vi "Waveplatecontrol_stepscan2.vi"() -> ()   [LabVIEW 2015]
uses:
  <vilib>/DAQmx/write.llb/DAQmx Write (Analog DBL 1Chan 1Samp).vi
  <vilib>/DAQmx/miscellaneous.llb/DAQmx Fill In Error Info.vi
  <vilib>/DAQmx/create/channels.llb/DAQmx Create Channel (AO-Voltage-Basic).vi
  <vilib>/Analysis/1siggen.llb/Ramp Pattern by Delta.vi
  subvi/Newport ESP301/Newport ESP301.lvlib
  <vilib>/Analysis/NI_AALBase.lvlib
panel:
  in  "StepSize":i32=128
  in  "ms2wait":u32
  in  "Boolean":bool
  out "a":waveform(dbl)(graph)={"t0"=timestamp(3620209335.8073797 s since 1904-01-01), "dt"=1.0, "Y"=[nan]}
  out "Waveform Chart":dbl(graph)=5.25341140860948
  out "x*y":dbl=nan
  in  "physical channels":tag="Dev3/ao1"
  out "DAC error":errorcluster
  out "ESP error":errorcluster={"status"=TRUE, "code"=-1073807343, "source"="VISA Open in Newport ESP301.lvlib:Initialize.vi->main002.vi"}
  out "run?":bool
  in  "set_vel":bool
  in  "velocity [fs/s]":dbl=667.128190396304
  in  "vel_mm":dbl caption="velocity [deg/s]"
  out "meas. velocity":dbl=nan
  in  "stop":bool
  out "output voltage":dbl=nan
  in  "start":bool
  in  "go2p1":bool
  out "position [mm]":dbl=nan
  in  "p2 [mm]":dbl=2.0
  in  "p1 [mm]":dbl
  in  "interpolate output":bool
  in  "Delta2 [fs]":dbl=6671.281903963041
  in  "Delta1 [fs]":dbl=-6671.281903963041
  in  "Reference [mm]":dbl=1.0
  in  "Axis (1)":i32=2 min=1 max=3
  in  "Serial Link (RS232)":enum16{"RS232", "USB"}(ring)
  in  "VISA resource name":refnum<visa-resource-name>="COM9"
  in  "main_close":bool
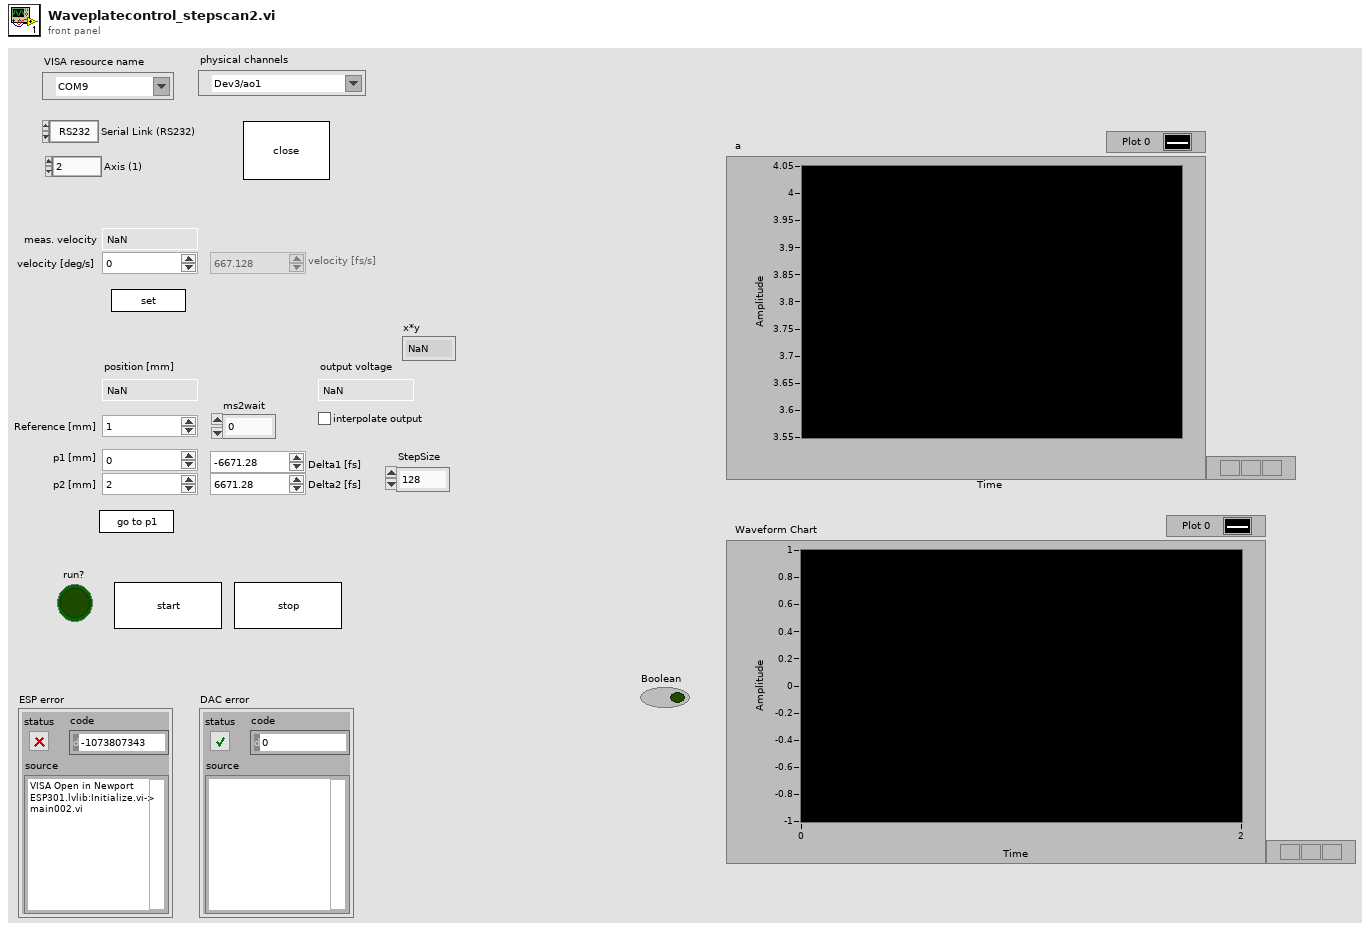
[diagram p1: front panel]
types:
  T1 = cluster{"dev1_data":refnum<queue>, "dev2_data":refnum<queue>}
  T2 = cluster{"dev1_cmd":refnum<queue>, "dev2_cmd":refnum<queue>}
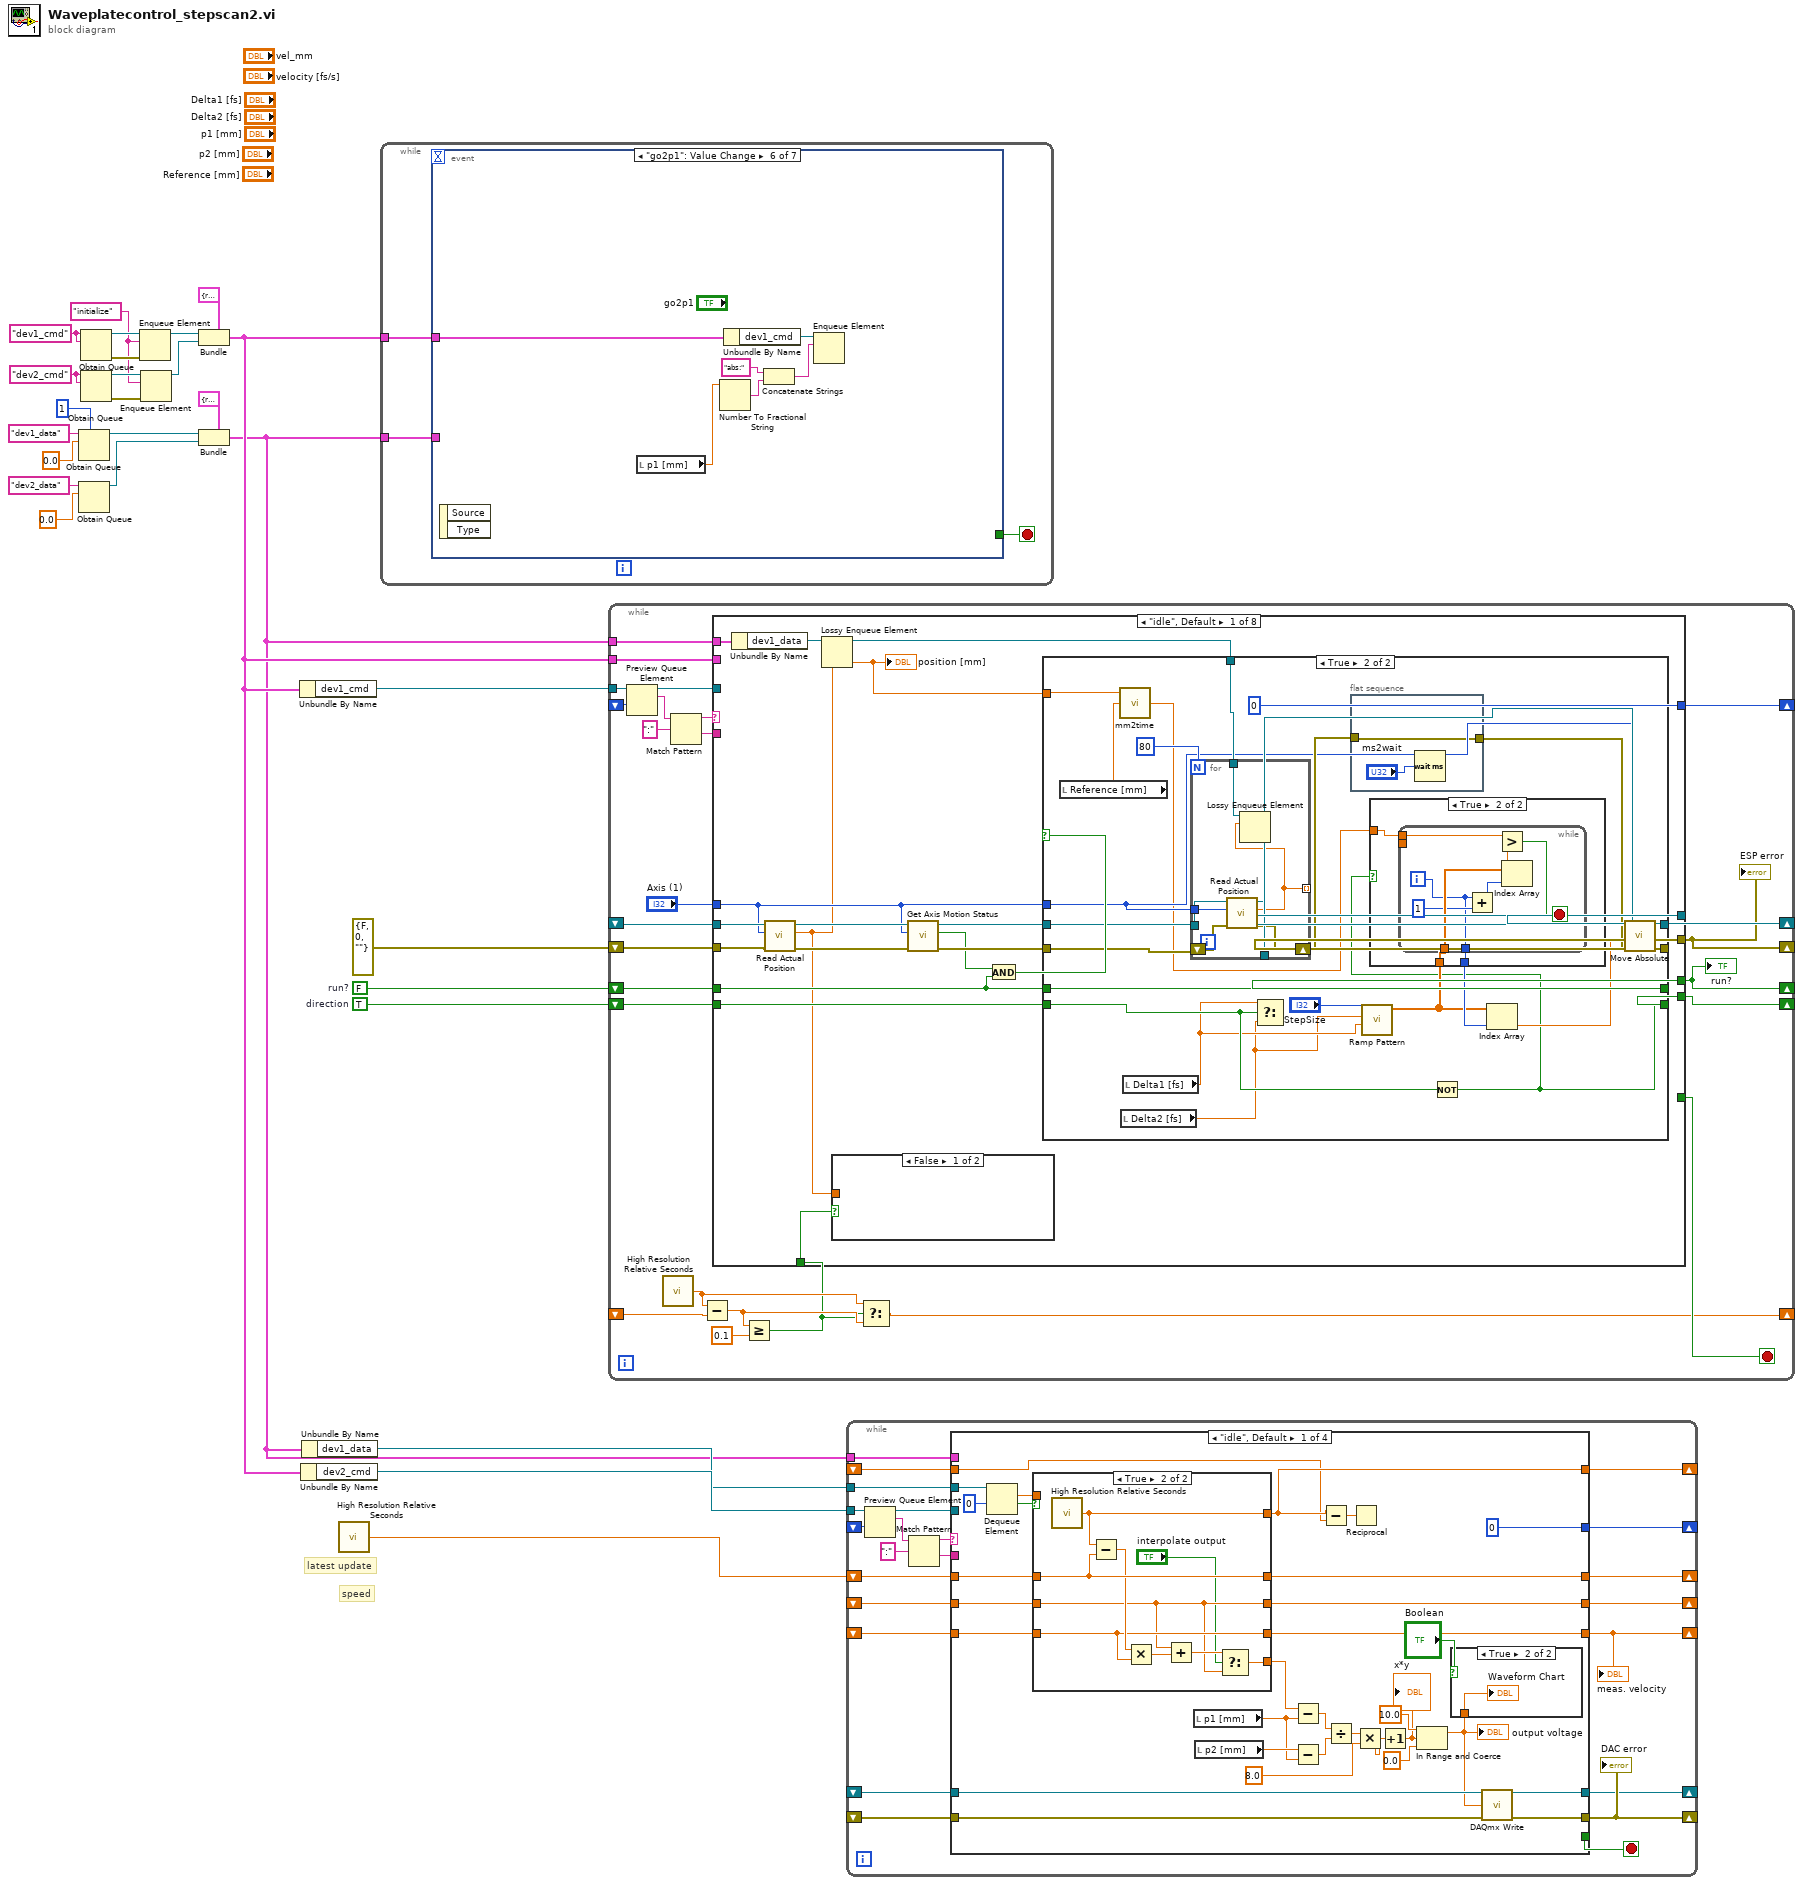
[diagram p0: block diagram]
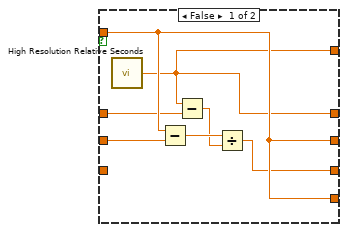
[diagram p3: hidden frame]
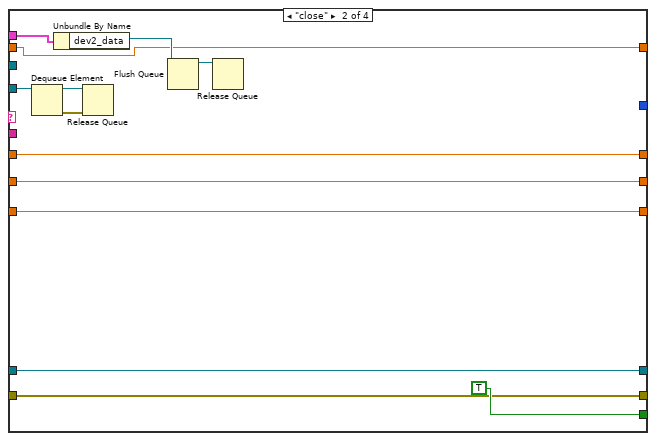
[diagram p4: hidden frame]
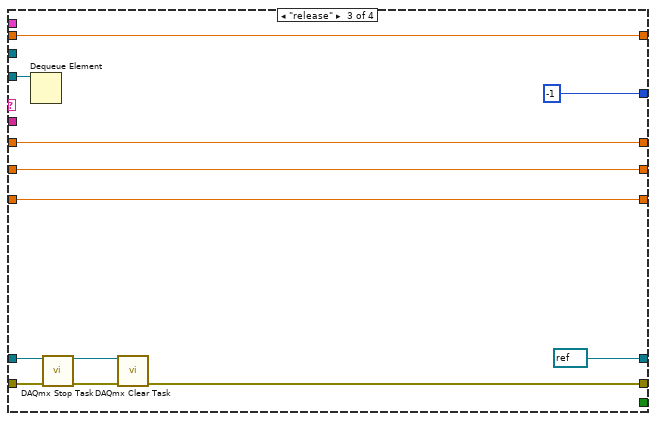
[diagram p5: hidden frame]
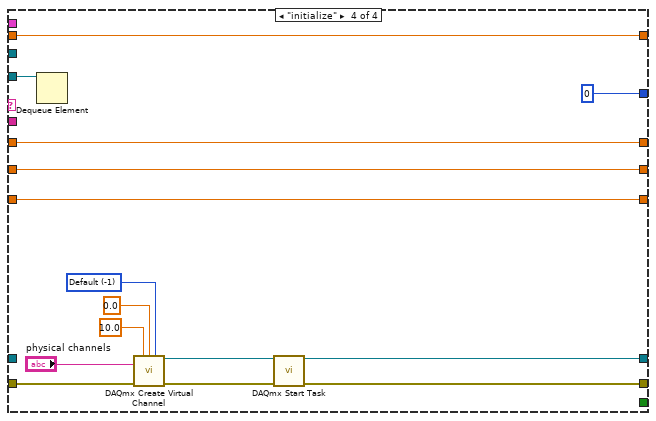
[diagram p6: hidden frame]
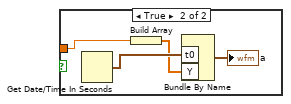
[diagram p7: hidden frame]
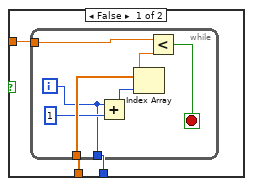
[diagram p9: hidden frame]
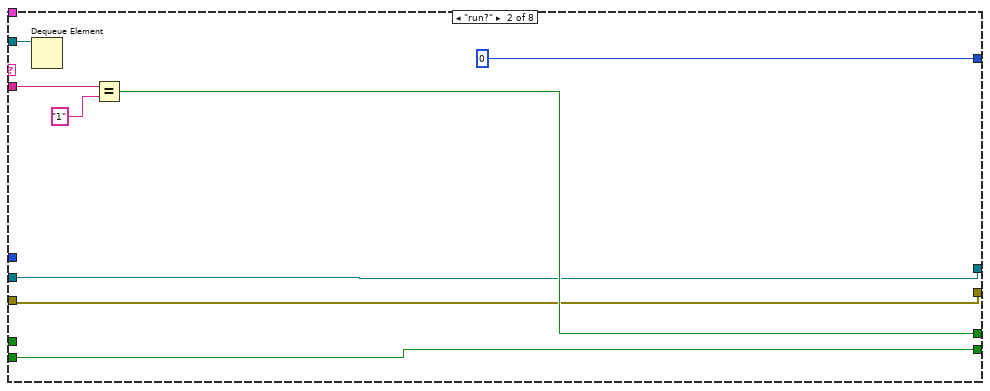
[diagram p10: hidden frame]
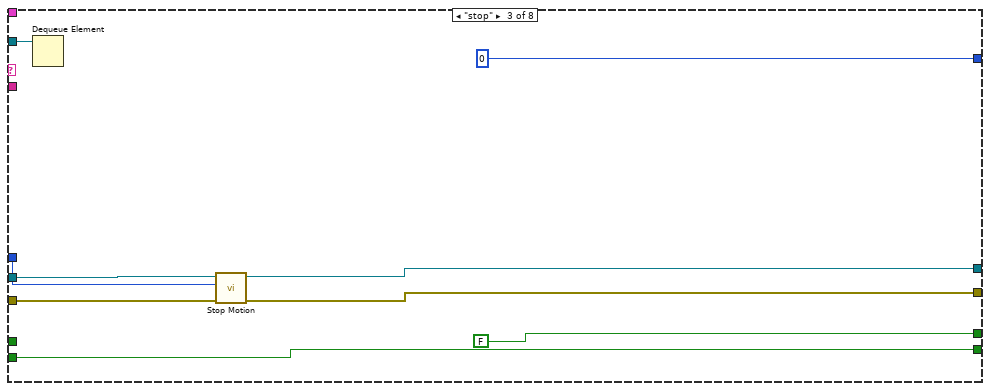
[diagram p11: hidden frame]
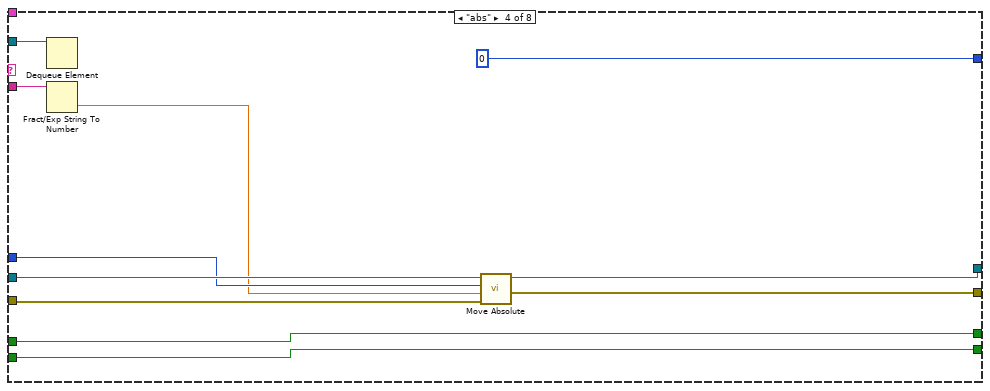
[diagram p12: hidden frame]
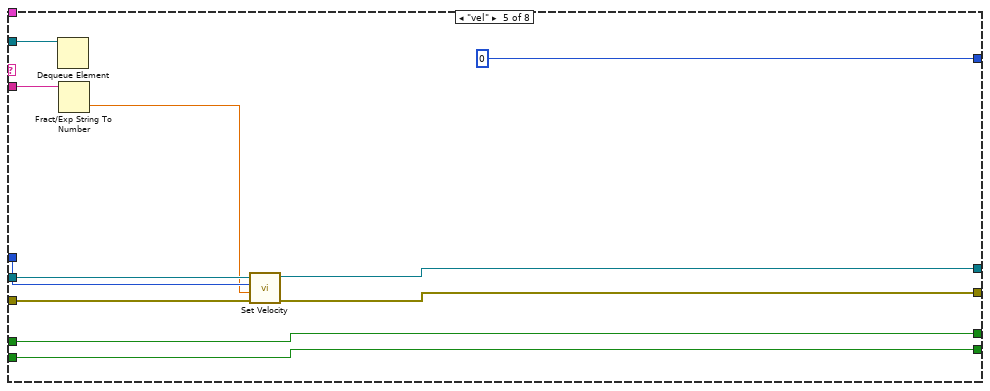
[diagram p13: hidden frame]
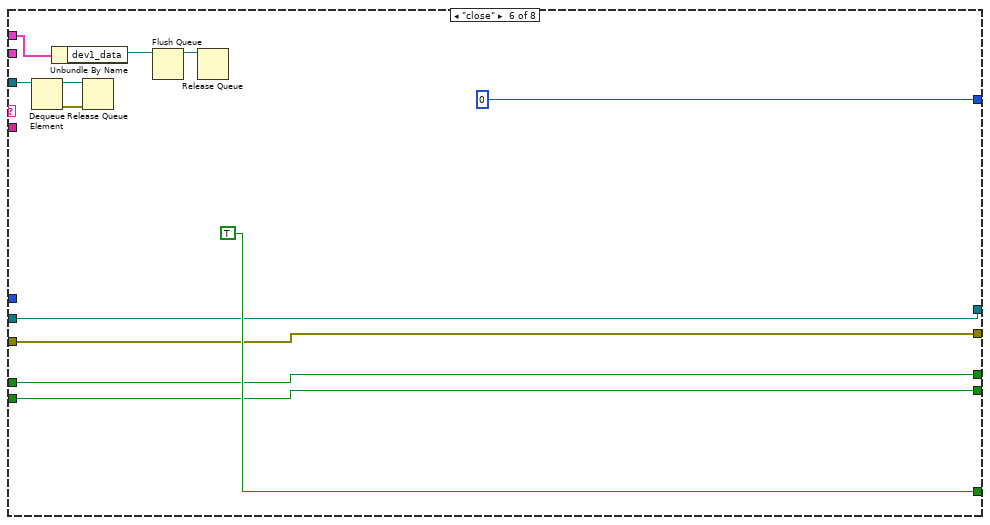
[diagram p14: hidden frame]
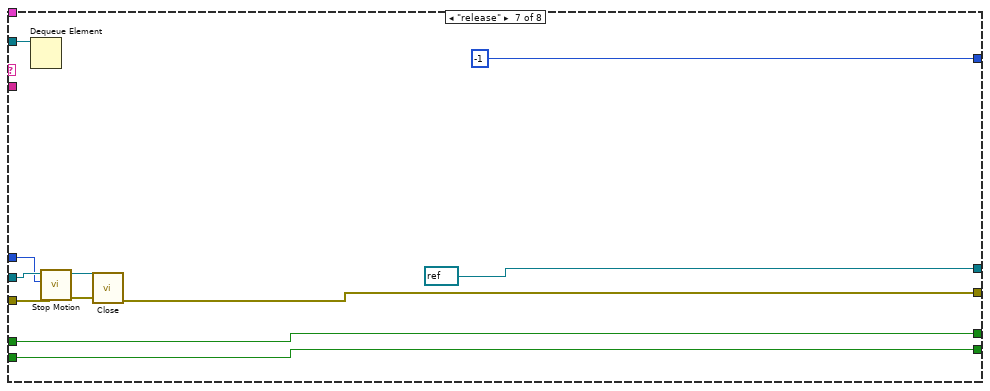
[diagram p15: hidden frame]
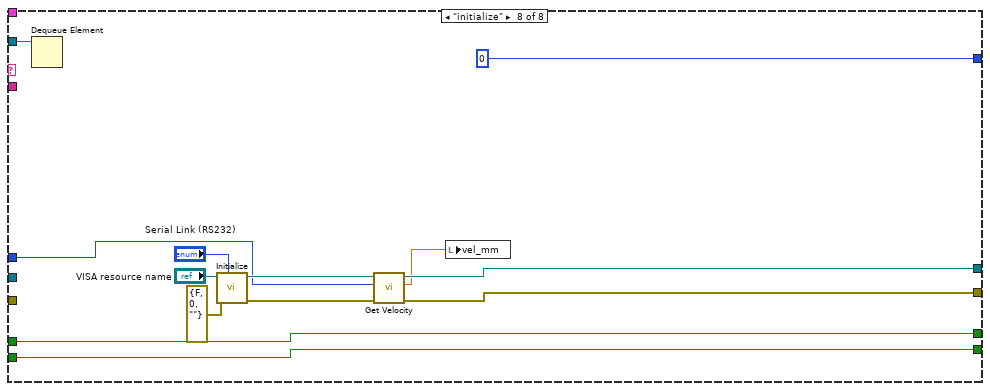
[diagram p16: hidden frame]
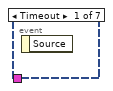
[diagram p17: hidden frame]
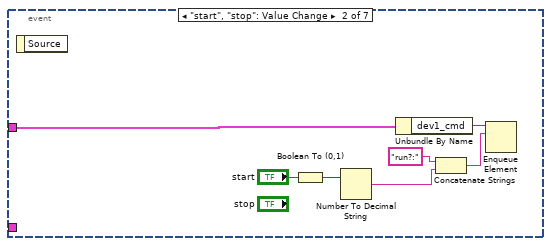
[diagram p18: hidden frame]
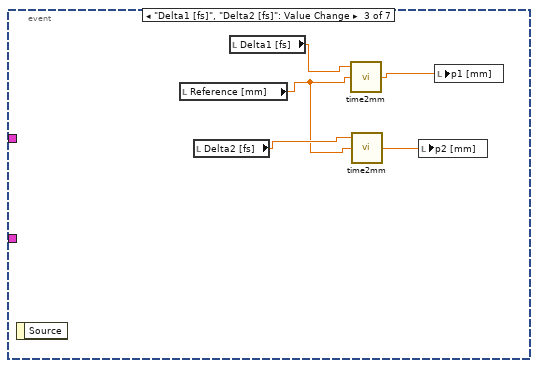
[diagram p19: hidden frame]
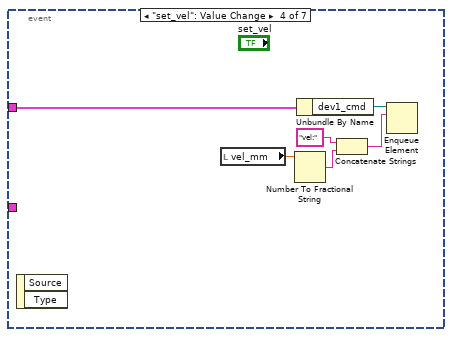
[diagram p20: hidden frame]
diagram:
  w1 = TRUE  # direction
  w4 = FALSE  # run?
  w15 = "dev2_cmd" ("name (unnamed)")
  w21 = "initialize" ("element")
  w16 = "dev1_cmd" ("name (unnamed)")
  # "speed"
  # "latest update"
  n1 = Obtain Queue(max queue size (-1, unlimited)=1, name (unnamed)="dev1_data", element data type=0.0) -> (queue out=w12:refnum<queue>)  [unwired: 2 in, 2 out]
  n2 = Obtain Queue(name (unnamed)="dev2_data", element data type=0.0) -> (queue out=w11:refnum<queue>)  [unwired: 3 in, 2 out]
  n3 = Obtain Queue(name (unnamed)=w16, element data type=w16) -> (queue out=w27:refnum<queue>, error out=w26:errorcluster)  [unwired: 3 in, 1 out]
  n4 = Obtain Queue(name (unnamed)=w15, element data type=w15) -> (queue out=w22:refnum<queue>, error out=w23:errorcluster)  [unwired: 3 in, 1 out]
  n5 = Enqueue Element(queue=w27, element=w21, error in (no error)=w26) -> (queue out=w24:refnum<queue>)  [unwired: 1 in, 2 out]
  n6 = Enqueue Element(queue=w22, element=w21, error in (no error)=w23) -> (queue out=w20:refnum<queue>)  [unwired: 1 in, 2 out]
  n7 = Bundle(cluster=T2 {"dev1_cmd"=refnum, "dev2_cmd"=refnum}, "dev1_cmd"=w24, "dev2_cmd"=w20) -> (w8:T2)
  n8 = Bundle(cluster=T1 {"dev1_data"=refnum, "dev2_data"=refnum}, "dev1_data"=w12, "dev2_data"=w11) -> (w2:T1)
  n9 = Unbundle By Name(w8) -> ("dev1_cmd"=w17:refnum<queue>)
  n10 = Unbundle By Name(w8) -> ("dev2_cmd"=w7:refnum<queue>)
  n11 = Unbundle By Name(w2) -> ("dev1_data"=w6:refnum<queue>)
  n12 = call <vilib>:"High Resolution Relative Seconds.vi"() -> ("relative seconds"=w5:dbl)
  n13 = while {
    tunnel: w8 -> [w30]
    tunnel: w2 -> [w29]
    stop <- w28 stop-if-true
    n14 = event shown="[5] \"go2p1\": Value Change" {
      selector: _ -> [_ _ _ _ _ _ _]
      dyn-events: _ -> [_ _ _ _ _ _ _]
      timeout: _ -> [_ _ _ _ _ _ _]
      tunnel: w30 -> [_ w34 _ w44 _ w62 w65]
      tunnel: w29 -> [_ _ _ _ _ _ _]
      tunnel: [_ _ _ _ _ _ TRUE] -> w28
      event Timeout {
        n15 = event-data() -> ()  [unwired: 1 in, 1 out]
      }
      event "start", "stop": Value Change {
        n16 = event-data() -> ()  [unwired: 1 in, 1 out]
        n17 = Boolean To (0,1)(Boolean="start") -> (0, 1=w32:i16)
        n18 = Number To Decimal String(number=w32) -> (decimal integer string=w31:string)  [unwired: 1 in]
        n19 = Unbundle By Name(w34) -> ("dev1_cmd"=w37:refnum<queue>)
        n20 = Concatenate Strings("run?:" ("string"), w31) -> (w36:string)
        n21 = Enqueue Element(queue=w37, element=w36) -> ()  [unwired: 2 in, 3 out]
      }
      event "Delta1 [fs]", "Delta2 [fs]": Value Change {
        n22 = event-data() -> ()  [unwired: 1 in, 1 out]
        n23 = local read "Reference [mm]"() -> (w39:dbl)
        n24 = local read "Delta2 [fs]"() -> (w40:dbl)
        n25 = local read "Delta1 [fs]"() -> (w42:dbl)
        n26 = call "time2mm.vi"("Offset (mm)"=w39, "time"=w42) -> ("position (mm)"=w41:dbl)  [unwired: 1 in]
        n27 = call "time2mm.vi"("Offset (mm)"=w39, "time"=w40) -> ("position (mm)"=w38:dbl)  [unwired: 1 in]
        n28 = local write "p2 [mm]"(w38) -> ()
        n29 = local write "p1 [mm]"(w41) -> ()
      }
      event "set_vel": Value Change {
        n30 = event-data() -> ()  [unwired: 1 in, 2 out]
        n31 = local read "vel_mm"() -> (w43:dbl)
        n32 = Number To Fractional String(number=w43) -> (F-format string=w47:string)  [unwired: 3 in]
        n33 = Unbundle By Name(w44) -> ("dev1_cmd"=w48:refnum<queue>)
        n34 = Concatenate Strings("vel:" ("string"), w47) -> (w46:string)
        n35 = Enqueue Element(queue=w48, element=w46) -> ()  [unwired: 2 in, 3 out]
      }
      event "p1 [mm]", "p2 [mm]", "Reference [mm]", "vel_mm": Value Change {
        n36 = event-data() -> ()  [unwired: 1 in, 2 out]
        n37 = local read "Reference [mm]"() -> (w54:dbl)
        n38 = local read "vel_mm"() -> (w51:dbl)
        n39 = local read "p1 [mm]"() -> (w55:dbl)
        n40 = local read "p2 [mm]"() -> (w56:dbl)
        n41 = call "mm2time.vi"("Offset (mm)"=0.0, "distance (mm)"=w51) -> ("time in fs"=w50:dbl)  [unwired: 1 in]
        n42 = call "mm2time.vi"("Offset (mm)"=w54, "distance (mm)"=w55) -> ("time in fs"=w52:dbl)  [unwired: 1 in]
        n43 = call "mm2time.vi"("Offset (mm)"=w54, "distance (mm)"=w56) -> ("time in fs"=w53:dbl)  [unwired: 1 in]
        n44 = local write "velocity [fs/s]"(w50) -> ()
        n45 = local write "Delta1 [fs]"(w52) -> ()
        n46 = local write "Delta2 [fs]"(w53) -> ()
      }
      event "go2p1": Value Change {
        n47 = event-data() -> ()  [unwired: 1 in, 2 out]
        n48 = local read "p1 [mm]"() -> (w57:dbl)
        n49 = Number To Fractional String(number=w57) -> (F-format string=w60:string)  [unwired: 3 in]
        n50 = Unbundle By Name(w62) -> ("dev1_cmd"=w61:refnum<queue>)
        n51 = Concatenate Strings("abs:" ("string"), w60) -> (w58:string)
        n52 = Enqueue Element(queue=w61, element=w58) -> ()  [unwired: 2 in, 3 out]
      }
      event "main_close": Value Change {
        n53 = event-data() -> ()  [unwired: 1 in, 1 out]
        n54 = Cluster To Array(cluster=w65) -> (array=w64:refnum<queue>[])
        n55 = for {
          tunnel: w64 -> [w70] mode=indexing
          n56 = Flush Queue(queue=w70) -> (queue out=w66:refnum<queue>)  [unwired: 1 in, 2 out]
          n57 = Enqueue Element(queue=w66, element="release") -> (queue out=w68:refnum<queue>)  [unwired: 2 in, 2 out]
          n58 = Enqueue Element(queue=w68, element="close") -> ()  [unwired: 2 in, 3 out]
        }
      }
    }
  }
  n59 = while {
    tunnel: w8 -> [w91]
    tunnel: w17 -> [w96]
    tunnel: w2 -> [w88]
    shift-right: [w86] -> _
    shift-left: _ -> [w87]
    shift-right: [w85] -> _
    shift-left: _ -> [w82]
    shift-right: [w84] -> _
    shift-left: errorcluster {"status"=FALSE, "code"=0, "source"=""} ("error out") -> [w83]
    shift-right: [w79] -> _
    shift-left: w4 -> [w80]
    shift-right: [w77] -> _
    shift-left: w1 -> [w78]
    shift-right: [w71] -> _
    shift-left: _ -> [w76]
    stop <- w89 stop-if-true
    n60 = Preview Queue Element(queue=w96, timeout in ms (-1)=w87) -> (queue out=w90:refnum<queue>, element=w95:string)  [unwired: 1 in, 2 out]
    n61 = call <vilib>:"High Resolution Relative Seconds.vi"() -> ("relative seconds"=w73:dbl)
    n62 = Match Pattern(string=w95, regular expression=":") -> (before substring=w93:string, after substring=w92:string)  [unwired: 1 in, 2 out]
    n63 = Subtract(x=w73, y=w76) -> (x-y=w74:dbl)
    n64 = Greater Or Equal?(x=w74, y=0.1) -> (x >= y?=w72:bool)
    n65 = case shown="\"idle\", Default" w93 {
      tunnel: w92 -> [_ w184 _ w203 w210 _ _ _]
      tunnel: w91 -> [_ _ _ _ _ _ _ _]
      tunnel: w90 -> [_ w182 w186 w204 w208 w227 w237 w247]
      tunnel: [_ _ _ _ _ TRUE _ _] -> w89
      tunnel: w88 -> [w116 _ _ _ _ w219 _ _]
      tunnel: [0 0 0 0 0 0 -1 0] -> w86
      tunnel: [w114 w177 w191 w200 w215 w223 refnum<visa-resource-name> refnum ("VISA resource name out") w243] -> w85
      tunnel: [w113 w178 w190 w199 w214 w222 w236 w242] -> w84
      tunnel: w83 -> [w111 w178 w192 w201 w213 w222 w232 _]
      tunnel: w82 -> [w112 w177 w193 w202 w212 w223 w229 _]
      tunnel: "Axis (1)" -> [w101 _ w189 w198 w211 _ w228 w244]
      tunnel: w80 -> [w99 _ _ w195 w206 w220 w234 w248]
      tunnel: [w108 w180 FALSE ("run?") w195 w206 w220 w234 w248] -> w79
      tunnel: w78 -> [w109 w179 w185 w194 w205 w216 w233 w239]
      tunnel: [w110 w179 w185 w194 w205 w216 w233 w239] -> w77
      tunnel: w72 -> [w107 _ _ _ _ _ _ _]
      frame "idle", Default {
        n66 = Unbundle By Name(w116) -> ("dev1_data"=w115:refnum<queue>)
        n67 = call "Read Actual Position.vi"("error in (no error)"=w111, "Axis (1)"=w101, "VISA resource name"=w112) -> ("error out"=w104:errorcluster, "Position (units)"=w97:dbl, "VISA resource name out"=w105:refnum<visa-resource-name>)  [unwired: 2 in]
        "position [mm]" <- w97
        n68 = Lossy Enqueue Element(queue=w115, element=w97) -> (queue out=w106:refnum<queue>)  [unwired: 1 in, 3 out]
        n69 = case shown="False" w107 {
          tunnel: w97 -> [_ w121]
          frame False {
          }
          frame True {
            n70 = Get Date/Time In Seconds() -> (seconds since 1Jan1904=w120:timestamp)
            n71 = Build Array(w121) -> (w119:dbl[])
            n72 = Bundle By Name("t0"=w120, "Y"=w119) -> (→"a":waveform(dbl))  [unwired: 1 in]
          }
        }
        n73 = call "Get Axis Motion Status.vi"("error in (no error)"=w104, "Axis (1)"=w101, "VISA resource name"=w105) -> ("error out"=w102:errorcluster, "Motion Done"=w100:bool, "VISA resource name out"=w103:refnum<visa-resource-name>)  [unwired: 2 in]
        n74 = And(x=w100, y=w99) -> (x .and. y?=w98:bool)
        n75 = case shown="True" w98 {
          tunnel: w103 -> [w125 w143]
          tunnel: w102 -> [w124 w144]
          tunnel: [w125 w141] -> w114
          tunnel: [w124 w140] -> w113
          tunnel: w101 -> [_ w137]
          tunnel: [w123 w129] -> w110
          tunnel: w109 -> [w123 w136]
          tunnel: w99 -> [w122 w147]
          tunnel: [w122 w147] -> w108
          tunnel: w106 -> [_ w146]
          tunnel: w97 -> [_ w128]
          frame False {
          }
          frame True {
            n76 = local read "Reference [mm]"() -> (w127:dbl)
            n77 = call "mm2time.vi"("Offset (mm)"=w127, "distance (mm)"=w128) -> ("time in fs"=w126:dbl)  [unwired: 1 in]
            n78 = local read "Delta2 [fs]"() -> (w134:dbl)
            n79 = local read "Delta1 [fs]"() -> (w135:dbl)
            n80 = for {
              N: 80 -> [_]
              tunnel: w143 -> [w176]
              tunnel: [w175] -> w139
              shift-right: [w171] -> w142
              shift-left: w144 -> [w174]
              tunnel: w137 -> [w173]
              tunnel: w146 -> [w172]
              tunnel: [w170] -> _ mode=indexing
              n81 = call "Read Actual Position.vi"("error in (no error)"=w174, "Axis (1)"=w173, "VISA resource name"=w176) -> ("error out"=w171:errorcluster, "Position (units)"=w170:dbl, "VISA resource name out"=w175:refnum<visa-resource-name>)  [unwired: 2 in]
              n82 = Lossy Enqueue Element(queue=w172, element=w170) -> ()  [unwired: 1 in, 4 out]
            }
            n83 = Select(t=w135, s=w136, f=w134) -> ()  [unwired: 1 out]
            n84 = flat-sequence {
              tunnel: w142 -> [w169]
              tunnel: [w169] -> w138
              frame #0 {
                n85 = Wait (ms)(milliseconds to wait="ms2wait") -> ()  [unwired: 1 out]
              }
            }
            n86 = call-poly <vilib>:"Ramp Pattern.vi"("start"=w135, "end"=w134, "delta"="StepSize") -> ("Ramp Pattern"=w130:dbl[])  [unwired: 6 in, 2 out]
            n87 = Not(x=w136) -> (.not. x?=w129:bool)
            n88 = case shown="True" w129 {
              tunnel: [w148 w160] -> w131
              tunnel: w130 -> [w149 w159]
              tunnel: w126 -> [w150 w158]
              frame False {
                n89 = while {
                  tunnel: w149 -> [w157]
                  tunnel: w150 -> [w153]
                  tunnel: [w154] -> w148
                  i -> [w154]
                  stop <- w151 stop-if-true
                  n90 = Add(x=w154, y=1) -> (x+y=w155:i32)
                  n91 = Index Array(array=w157, index=w155) -> (element=w152:dbl)
                  n92 = Less?(x=w153, y=w152) -> (x < y?=w151:bool)
                }
              }
              frame True {
                n93 = while {
                  tunnel: w159 -> [w167]
                  tunnel: [w163] -> _
                  tunnel: w158 -> [w163]
                  tunnel: [w161] -> w160
                  i -> [w161]
                  stop <- w162 stop-if-true
                  n94 = Add(x=w161, y=1) -> (x+y=w165:i32)
                  n95 = Index Array(array=w167, index=w165) -> (element=w164:dbl)
                  n96 = Greater?(x=w163, y=w164) -> (0:w162:bool)
                }
              }
            }
            n97 = Index Array(array=w130, index=w131) -> (element=w132:dbl)
            n98 = call "Move Absolute.vi"("error in (no error)"=w138, "Position (0 units)"=w132, "Axis (1)"=w137, "VISA resource name"=w139) -> ("error out"=w140:errorcluster, "VISA resource name out"=w141:refnum<visa-resource-name>)  [unwired: 2 in]
          }
        }
      }
      frame "run?" {
        n99 = Dequeue Element(queue=w182) -> ()  [unwired: 2 in, 4 out]
        n100 = Equal?(x=w184, y="1") -> (x = y?=w180:bool)
      }
      frame "stop" {
        n101 = Dequeue Element(queue=w186) -> ()  [unwired: 2 in, 4 out]
        n102 = call "Stop Motion.vi"("error in (no error)"=w192, "Axis (1)"=w189, "VISA resource name"=w193) -> ("error out"=w190:errorcluster, "VISA resource name out"=w191:refnum<visa-resource-name>)  [unwired: 3 in]
      }
      frame "abs" {
        n103 = Dequeue Element(queue=w204) -> ()  [unwired: 2 in, 4 out]
        n104 = Fract/Exp String To Number(string=w203) -> (number=w197:dbl)  [unwired: 3 in, 1 out]
        n105 = call "Move Absolute.vi"("error in (no error)"=w201, "Position (0 units)"=w197, "Axis (1)"=w198, "VISA resource name"=w202) -> ("error out"=w199:errorcluster, "VISA resource name out"=w200:refnum<visa-resource-name>)  [unwired: 2 in]
      }
      frame "vel" {
        n106 = Dequeue Element(queue=w208) -> ()  [unwired: 2 in, 4 out]
        n107 = Fract/Exp String To Number(string=w210) -> (number=w209:dbl)  [unwired: 3 in, 1 out]
        n108 = call "Set Velocity.vi"("error in (no error)"=w213, "Velocity (units/s)"=w209, "Axis (1)"=w211, "VISA resource name"=w212) -> ("error out"=w214:errorcluster, "VISA resource name out"=w215:refnum<visa-resource-name>)  [unwired: 2 in]
      }
      frame "close" {
        n109 = Dequeue Element(queue=w227) -> (queue out=w226:refnum<queue>, error out=w225:errorcluster)  [unwired: 2 in, 2 out]
        n110 = Unbundle By Name(w219) -> ("dev1_data"=w217:refnum<queue>)
        n111 = Release Queue(queue=w226, error in (no error)=w225) -> ()  [unwired: 1 in, 3 out]
        n112 = Flush Queue(queue=w217) -> (queue out=w218:refnum<queue>)  [unwired: 1 in, 2 out]
        n113 = Release Queue(queue=w218) -> ()  [unwired: 2 in, 3 out]
      }
      frame "release" {
        n114 = Dequeue Element(queue=w237) -> ()  [unwired: 2 in, 4 out]
        n115 = call "Stop Motion.vi"("error in (no error)"=w232, "Axis (1)"=w228, "VISA resource name"=w229) -> ("error out"=w231:errorcluster, "VISA resource name out"=w230:refnum<visa-resource-name>)  [unwired: 3 in]
        n116 = call "Close.vi"("error in (no error)"=w231, "VISA resource name"=w230) -> ("error out"=w236:errorcluster)  [unwired: 9 in]
      }
      frame "initialize" {
        n117 = Dequeue Element(queue=w247) -> ()  [unwired: 2 in, 4 out]
        n118 = call "Initialize.vi"("VISA resource name"="VISA resource name", "error in (no error)"=errorcluster {"status"=FALSE, "code"=0, "source"=""}, "Serial Link (RS232)"="Serial Link (RS232)") -> ("VISA resource name out"=w246:refnum<visa-resource-name>, "error out"=w245:errorcluster)  [unwired: 6 in]
        n119 = call "Get Velocity.vi"("error in (no error)"=w245, "Axis (1)"=w244, "VISA resource name"=w246) -> ("error out"=w242:errorcluster, "Velocity (units/s)"=w241:dbl, "VISA resource name out"=w243:refnum<visa-resource-name>)  [unwired: 2 in]
        n120 = local write "vel_mm"(w241) -> ()
      }
    }
    "run?" <- w79
    "ESP error" <- w84
    n121 = Select(t=w73, s=w72, f=w74) -> (s? t:f=w71:dbl)
  }
  n122 = while {
    shift-right: [w267] -> _
    shift-left: _ -> [w268]
    shift-right: [w266] -> _
    shift-left: _ -> [w265]
    tunnel: w7 -> [w264]
    shift-right: [w263] -> _
    shift-left: _ -> [w262]
    tunnel: w6 -> [w261]
    shift-right: [w260] -> _
    shift-left: _ -> [w257]
    shift-right: [w259] -> _
    shift-left: w5 -> [w258]
    shift-right: [w252] -> _
    shift-left: _ -> [w256]
    tunnel: w2 -> [w255]
    shift-right: [w254] -> _
    shift-left: _ -> [w253]
    stop <- w269 stop-if-true
    n123 = Preview Queue Element(queue=w264, timeout in ms (-1)=w268) -> (queue out=w270:refnum<queue>, element=w274:string)  [unwired: 1 in, 2 out]
    n124 = Match Pattern(string=w274, regular expression=":") -> (before substring=w272:string, after substring=w271:string)  [unwired: 1 in, 2 out]
    n125 = case shown="\"idle\", Default" w272 {
      tunnel: w271 -> [_ _ _ _]
      tunnel: w270 -> [_ w335 w346 w354]
      tunnel: [_ TRUE _ _] -> w269
      tunnel: [0 _ -1 0] -> w267
      tunnel: [w301 w331 w345 w355] -> w266
      tunnel: w265 -> [w299 w331 w342 w362]
      tunnel: [w302 w330 refnum<k21> refnum ("task out") w356] -> w263
      tunnel: w262 -> [w300 w330 w343 _]
      tunnel: w261 -> [w303 _ _ _]
      tunnel: [w297 w328 w338 w351] -> w260
      tunnel: [w296 w329 w339 w352] -> w259
      tunnel: w258 -> [w294 w329 w339 w352]
      tunnel: w257 -> [w295 w328 w338 w351]
      tunnel: [w293 w327 w337 w350] -> w252
      tunnel: w256 -> [w292 w327 w337 w350]
      tunnel: w255 -> [_ w324 _ _]
      tunnel: [w281 w323 w336 w348] -> w254
      tunnel: w253 -> [w280 w323 w336 w348]
      frame "idle", Default {
        n126 = Dequeue Element(queue=w303, timeout in ms (-1)=0) -> (element=w298:dbl, timed out?=w282:bool)  [unwired: 1 in, 2 out]
        n127 = case shown="True" w282 {
          tunnel: w298 -> [w313 _]
          tunnel: [w313 w315] -> w291
          tunnel: [w313 w317] -> w297
          tunnel: [w307 w322] -> w296
          tunnel: w295 -> [w312 w317]
          tunnel: w294 -> [w311 w322]
          tunnel: [w308 w319] -> w293
          tunnel: w292 -> [_ w319]
          tunnel: [w307 w314] -> w281
          frame False {
            n128 = call <vilib>:"High Resolution Relative Seconds.vi"() -> ("relative seconds"=w307:dbl)
            n129 = Subtract(x=w313, y=w312) -> (x-y=w310:dbl)
            n130 = Subtract(x=w307, y=w311) -> (x-y=w309:dbl)
            n131 = Divide(x=w310, y=w309) -> (x/y=w308:dbl)
          }
          frame True {
            n132 = call <vilib>:"High Resolution Relative Seconds.vi"() -> ("relative seconds"=w314:dbl)
            n133 = Subtract(x=w314, y=w322) -> (x-y=w321:dbl)
            n134 = Multiply(x=w321, y=w319) -> (x*y=w320:dbl)
            n135 = Add(x=w317, y=w320) -> (x+y=w318:dbl)
            n136 = Select(t=w318, s="interpolate output", f=w317) -> (s? t:f=w315:dbl)
          }
        }
        n137 = local read "p1 [mm]"() -> (w289:dbl)
        n138 = local read "p2 [mm]"() -> (w290:dbl)
        n139 = Subtract(x=w291, y=w289) -> (x-y=w288:dbl)
        n140 = Subtract(x=w290, y=w289) -> (x-y=w287:dbl)
        n141 = Subtract(x=w281, y=w280) -> (x-y=w279:dbl)
        n142 = Divide(x=w288, y=w287) -> (x/y=w286:dbl)
        n143 = Reciprocal(x=w279) -> ()  [unwired: 1 out]
        n144 = Multiply(x=w286, y=8.0) -> (x*y=w277:dbl)
        n145 = Increment(x=w277) -> (x+1=w276:dbl)
        "x*y" <- w276
        n146 = In Range and Coerce(upper limit=10.0, x=w276, lower limit=0.0) -> (coerced(x)=w278:dbl)  [unwired: 1 out]
        "output voltage" <- w278
        n147 = case shown="True" "Boolean" {
          tunnel: w278 -> [_ w306]
          frame False {
          }
          frame True {
            "Waveform Chart" <- w306
          }
        }
        n148 = call-poly <vilib>:"DAQmx Write.vi"("task/channels in"=w300, "data"=w278, "error in"=w299) -> ("task out"=w302:refnum<k21>, "error out"=w301:errorcluster)  [unwired: 10 in, 1 out]
      }
      frame "close" {
        n149 = Dequeue Element(queue=w335) -> (queue out=w334:refnum<queue>, error out=w333:errorcluster)  [unwired: 2 in, 2 out]
        n150 = Unbundle By Name(w324) -> ("dev2_data"=w325:refnum<queue>)
        n151 = Release Queue(queue=w334, error in (no error)=w333) -> ()  [unwired: 1 in, 3 out]
        n152 = Flush Queue(queue=w325) -> (queue out=w326:refnum<queue>)  [unwired: 1 in, 2 out]
        n153 = Release Queue(queue=w326) -> ()  [unwired: 2 in, 3 out]
      }
      frame "release" {
        n154 = Dequeue Element(queue=w346) -> ()  [unwired: 2 in, 4 out]
        n155 = call <vilib>:"DAQmx Stop Task.vi"("task/channels in"=w343, "error in"=w342) -> ("task out"=w341:refnum<k21>, "error out"=w340:errorcluster)  [unwired: 12 in]
        n156 = call <vilib>:"DAQmx Clear Task.vi"("task in"=w341, "error in"=w340) -> ("error out"=w345:errorcluster)  [unwired: 13 in]
      }
      frame "initialize" {
        w359 = -1 items=["Default"=-1, "RSE"=10083, "Differential"=10106, "Pseudodifferential"=12529] ("output terminal configuration")
        n157 = Dequeue Element(queue=w354) -> ()  [unwired: 2 in, 4 out]
        n158 = call-poly <vilib>:"DAQmx Create Virtual Channel.vi"("maximum value"=10.0, "minimum value"=0.0, "output terminal configuration"=w359, "physical channels"="physical channels", "error in"=w362) -> ("task out"=w358:refnum<k21>, "error out"=w357:errorcluster)  [unwired: 9 in]
        n159 = call <vilib>:"DAQmx Start Task.vi"("task/channels in"=w358, "error in"=w357) -> ("task out"=w356:refnum<k21>, "error out"=w355:errorcluster)  [unwired: 12 in]
      }
    }
    "meas. velocity" <- w252
    "DAC error" <- w266
  }
